vi "GPS Sort Waypoint List.vi"(10 "Current co-ordinate":T1 {"Longitude" format="%#_14g"; "Latitude" format="%#_14g"}, 11 "Unsorted Waypoint List":T1[](array[typedef]) {"Longitude" format="%#_14g"; "Latitude" format="%#_14g"}) -> (3 "Sorted Waypoints":T1[](array[typedef]) {"Longitude" format="%#_14g"; "Latitude" format="%#_14g"})   [LabVIEW 2009]
uses:
  TypeDefs/Sensor TypeDefs/GPS Data.ctl
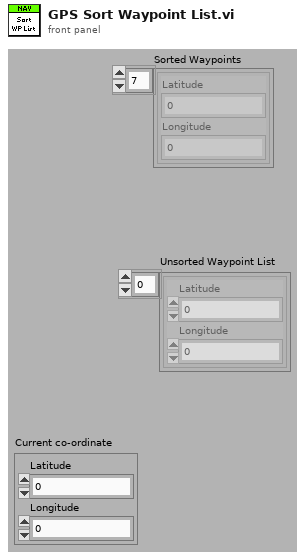
[diagram p1: front panel]
types:
  T1 = typedef "GPS Data.ctl" = cluster{"Latitude":dbl, "Longitude":dbl}
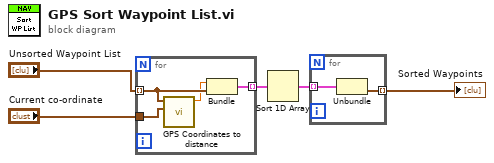
[diagram p0: block diagram]
diagram:
  n1 = for {
    tunnel: "Unsorted Waypoint List" -> [w8] mode=indexing
    tunnel: "Current co-ordinate" -> [w7]
    tunnel: [w9] -> w2 mode=indexing
    n2 = call "GPS Coordinates to distance.vi"("GPS Co-ordinate 2"=w7, "GPS Co-ordinate 1"=w8) -> ("Distance"=w6:dbl)  [unwired: 9 in]
    n3 = Bundle("Distance"=w6, "GPS Co-ordinate"=w8) -> (w9:cluster{"Distance":dbl, "GPS Co-ordinate":T1})  [unwired: 1 in]
  }
  n4 = Sort 1D Array(array=w2) -> (sorted array=w1:cluster{"Distance":dbl, "GPS Co-ordinate":T1}[])
  n5 = for {
    tunnel: w1 -> [w11] mode=indexing
    tunnel: [w10] -> w5 mode=indexing
    n6 = Unbundle(w11) -> ("GPS Co-ordinate"=w10:T1)  [unwired: 1 out]
  }
  "Sorted Waypoints" <- w5
